vi "Get Name.vi"(11 "Linked List Definition in":refnum<class "Linked List Definition.lvclass">) -> (1 "I am Root?":bool, 2 "Unique ID":string, 3 "Name":string)   [LabVIEW 2020, in "Linked Lists.lvlib" / "Linked List Definition.lvclass"]
uses:
  <vilib>/gpm_packages/@cs/linked-list/Source/Linked List/Linked List Definition/Linked List Definition.lvclass
  <vilib>/gpm_packages/@cs/linked-list/Source/Linked List/Linked List Definition/Linked List Definition.lvclass/Linked List Definition.ctl
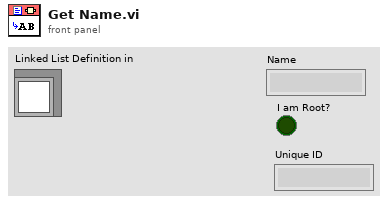
[diagram p1: front panel]
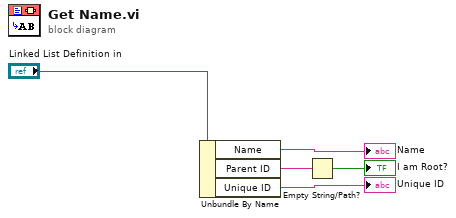
[diagram p0: block diagram]
diagram:
  n1 = Unbundle By Name("Linked List Definition in") -> ("Name"=→"Name":string, "Parent ID"=w3:string, "Unique ID"=→"Unique ID":string)
  n2 = Empty String/Path?(string/path=w3) -> (empty?=→"I am Root?":bool)
